vi "DPT TC Panel Read.vi"(10 "all rows":string[][](array[string]), 11 "TC Panel 1":T1[][](array[typedef])=[[{"Label"="RDB F", "Record"=TRUE, "Index"=0, "Channel"=""}, {"Label"="Room Ambient(F)", "Record"=TRUE, "Index"=0, "Channel"=""}, {"Label"="Tscale", "Record"=TRUE, "Index"=0, "Channel"=""}, {"Label"="", "Record"=FALSE, "Index"=0, "Channel"=""}, {"Label"="", "Record"=FALSE, "Index"=0, "Channel"=""}, {"Label"="", "Record"=FALSE, "Index"=0, "Channel"=""}], [{"Label"="", "Record"=FALSE, "Index"=0, "Channel"=""}, {"Label"="", "Record"=FALSE, "Index"=0, "Channel"=""}, {"Label"="", "Record"=FALSE, "Index"=0, "Channel"=""}, {"Label"="", "Record"=FALSE, "Index"=0, "Channel"=""}, {"Label"="", "Record"=FALSE, "Index"=0, "Channel"=""}, {"Label"="", "Record"=FALSE, "Index"=0, "Channel"=""}], [{"Label"="", "Record"=FALSE, "Index"=0, "Channel"=""}, {"Label"="", "Record"=FALSE, "Index"=0, "Channel"=""}, {"Label"="", "Record"=FALSE, "Index"=0, "Channel"=""}, {"Label"="", "Record"=FALSE, "Index"=0, "Channel"=""}, {"Label"="", "Record"=FALSE, "Index"=0, "Channel"=""}, {"Label"="", "Record"=FALSE, "Index"=0, "Channel"=""}]]) -> (3 "TC Panel 2":T1[][](array[typedef])=[[{"Label"="RDB F", "Record"=TRUE, "Index"=0, "Channel"=""}, {"Label"="Room Ambient(F)", "Record"=TRUE, "Index"=0, "Channel"=""}, {"Label"="Tscale", "Record"=TRUE, "Index"=0, "Channel"=""}, {"Label"="", "Record"=FALSE, "Index"=0, "Channel"=""}, {"Label"="", "Record"=FALSE, "Index"=0, "Channel"=""}, {"Label"="", "Record"=FALSE, "Index"=0, "Channel"=""}], [{"Label"="", "Record"=FALSE, "Index"=0, "Channel"=""}, {"Label"="", "Record"=FALSE, "Index"=0, "Channel"=""}, {"Label"="", "Record"=FALSE, "Index"=0, "Channel"=""}, {"Label"="", "Record"=FALSE, "Index"=0, "Channel"=""}, {"Label"="", "Record"=FALSE, "Index"=0, "Channel"=""}, {"Label"="", "Record"=FALSE, "Index"=0, "Channel"=""}], [{"Label"="", "Record"=FALSE, "Index"=0, "Channel"=""}, {"Label"="", "Record"=FALSE, "Index"=0, "Channel"=""}, {"Label"="", "Record"=FALSE, "Index"=0, "Channel"=""}, {"Label"="", "Record"=FALSE, "Index"=0, "Channel"=""}, {"Label"="", "Record"=FALSE, "Index"=0, "Channel"=""}, {"Label"="", "Record"=FALSE, "Index"=0, "Channel"=""}]])   [LabVIEW 2016]
doc: "Read file contents and place information into respective panels."
uses:
  Type Definitions/DPT Channel Label.ctl
  Utility/Custom Pallet Controls/Custom Pallet String.ctl
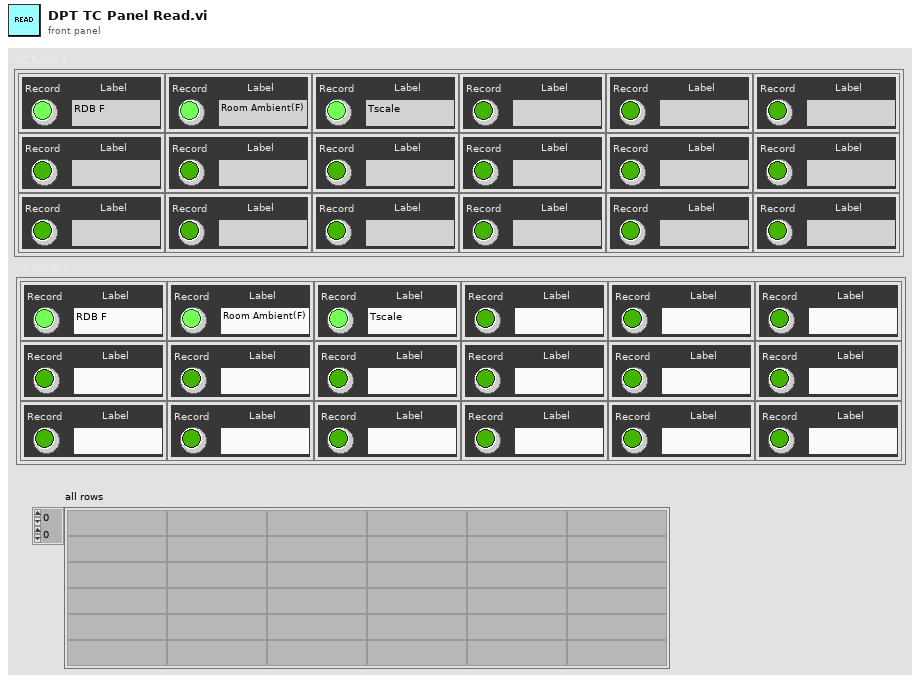
[diagram p1: front panel]
types:
  T1 = typedef "DPT Channel Label.ctl" = cluster{"Label":T2, "Record":bool, "Index":u32, "Channel":string}
  T2 = typedef "Custom Pallet String.ctl" = string
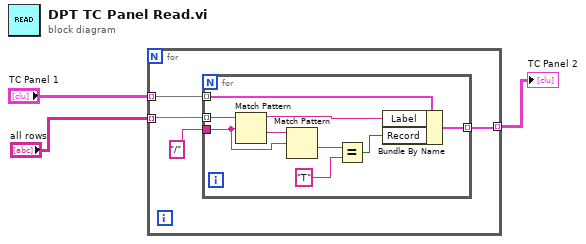
[diagram p0: block diagram]
diagram:
  n1 = for {
    tunnel: "TC Panel 1" -> [w6] mode=indexing
    tunnel: "all rows" -> [w5] mode=indexing
    tunnel: [w4] -> w1 mode=indexing
    n2 = for {
      tunnel: w6 -> [w15] mode=indexing
      tunnel: w5 -> [w16] mode=indexing
      tunnel: [w13] -> w4 mode=indexing
      tunnel: "/" ("regular expression") -> [w8]
      n3 = Match Pattern(string=w16, regular expression=w8) -> (before substring=w14:string, after substring=w12:string)  [unwired: 1 in, 2 out]
      n4 = Match Pattern(string=w12, regular expression=w8) -> (after substring=w11:string)  [unwired: 1 in, 3 out]
      n5 = Equal?(x=w11, y="T") -> (x = y?=w9:bool)
      n6 = Bundle By Name(cluster=w15, "Label"=w14, "Record"=w9) -> (w13:T1)
    }
  }
  "TC Panel 2" <- w1
